vi "EdgeDetect_Camera.vi"(5 "did":string="aa5f5cb08903b53f224287e0", 7 "wid":string="e1f73355bdbd9a727fdd999e", 9 "eid":string, 11 "Scaling Factor":dbl) -> (4 "Device Out":T2, 6 "Comm":T1, 8 "image 2":picture, 15 "error out":errorcluster)   [LabVIEW 2019]
uses:
  <userlib>/Onshape/_SubVI/Cluster.ctl
  <userlib>/IoT Devices/_subVIs/HTTPComm.ctl
  <userlib>/Onshape/_SubVI/z did wid and eid.vi
  <userlib>/OnshapeFeatureFunctions/Onshape Feature Funcrions/_SubVI/FS Sketch Polyline.vi
  <userlib>/OnshapeFeatureFunctions/Onshape Feature Funcrions/_SubVI/FS Operation Extrude.vi
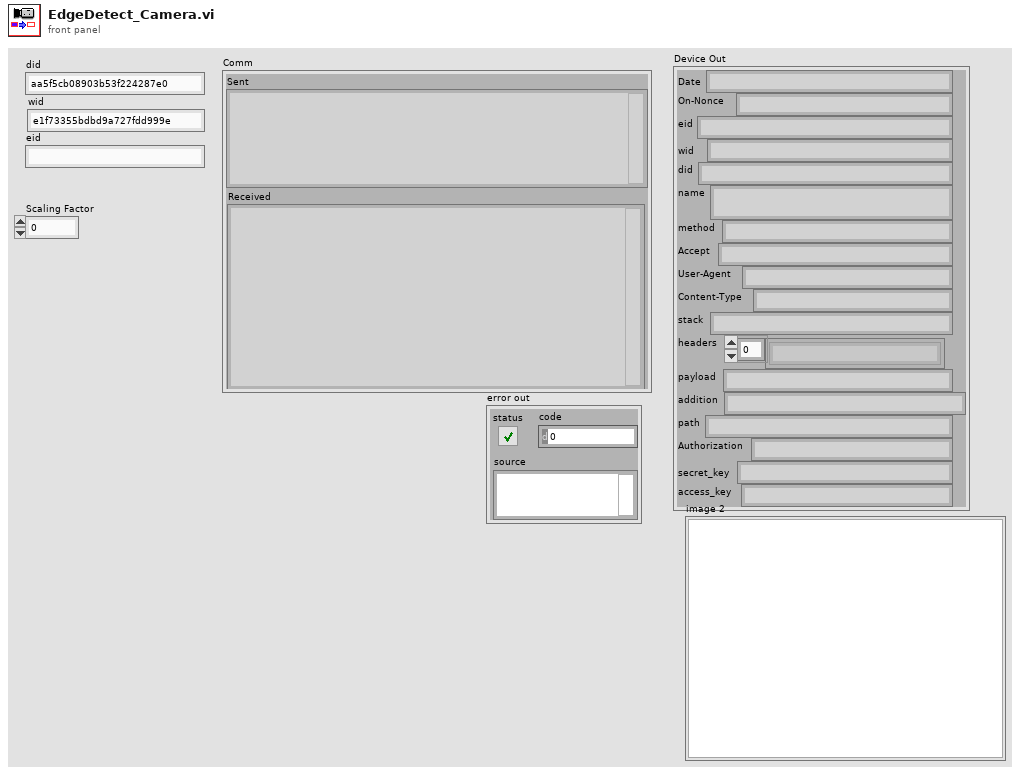
[diagram p1: front panel]
types:
  T1 = typedef "HTTPComm.ctl" = cluster{"url":string, "sent headers":string, "sent body":string, "headers":string, "body":string, "Sent":string, "Received":string}
  T2 = typedef "Cluster.ctl" = cluster{"Date":string, "On-Nonce":string, "eid":string, "wid":string, "did":string, "name":string, "method":string, "Accept":string, "User-Agent":string, "Content-Type":string, "stack":string, "headers":string[], "payload":string, "addition":string, "path":string, "Authorization":string, "secret_key":string, "access_key":string}
  T3 = typedef "QT_Image.ctl" = cluster{"Width":i32, "Height":i32, "Depth":i32, "data":u8[], "Compressed data":u8[], "Color table":u32[], "Duration":i32, "Options":i32, "Timestamp":i32, "ID":i32, "Reserved":i32, "Dialogs":u32}
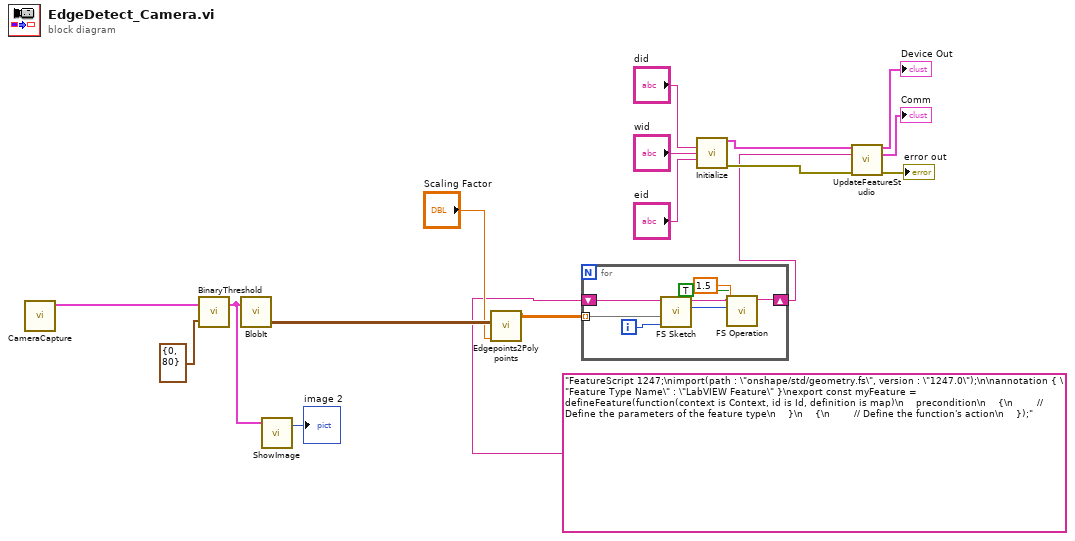
[diagram p0: block diagram]
diagram:
  n1 = call <userlib>:"CameraCapture.vi"() -> ("Image  out"=w4:T3)  [unwired: 11 in]
  n2 = call <userlib>:"BinaryThreshold.vi"("threshold"=cluster{u8, u8} {0, 80}, "Image In"=w4) -> ("Image Out"=w6:T3)  [unwired: 1 in]
  n3 = call <userlib>:"BlobIt.vi"("Image in"=w6) -> ("Array 2"=w17:cluster{"Row":i32, "Col":i32}[][])  [unwired: 1 in, 2 out]
  n4 = call <userlib>:"ShowImage.vi"("Image"=w6) -> ("image"=→"image 2":picture)  [unwired: 2 in, 1 out]
  n5 = call <userlib>:"Edgepoints2Polypoints.vi"("Scaling Factor"="Scaling Factor", "Edgepoints In"=w17) -> ("Polyline Out"=w2:dbl[][][])  [unwired: 9 in]
  n6 = for {
    tunnel: w2 -> [w24] mode=indexing
    shift-right: [w21] -> w1
    shift-left: "FeatureScript 1247;\nimport(path : \"onshape/std/geometry.fs\", version : \"1247.0\");\n\nannotation { \"Feature Type Name\" : \"LabVIEW Feature\" }\nexport const myFeature = defineFeature(function(context is Context, id is Id, definition is map)\n    precondition\n    {\n        // Define the parameters of the feature type\n    }\n    {\n        // Define the function's action\n    });" ("Feature In") -> [w23]
    i -> [w18]
    n7 = call-poly <userlib>:"FS Sketch.vi"("Sketch #"=w18, "Polyline Points"=w24, "Feature In"=w23) -> ("Feature Out"=w22:string)  [unwired: 8 in]
    n8 = call-poly <userlib>:"FS Operation.vi"("Ignore Inner Loops?"=TRUE, "Extrude Depth"=1.5, "Sketch # to Extrude"=w18, "Feature In"=w22) -> ("Feature Out"=w21:string)  [unwired: 7 in]
  }
  n9 = call-poly <userlib>:"Initialize.vi"("did"="did", "wid"="wid", "eid"="eid") -> ("Device Out"=w13:T2, "error out"=w7:errorcluster)  [unwired: 11 in]
  n10 = call <userlib>:"UpdateFeatureStudio.vi"("Device In"=w13, "FeatureScript"=w1, "error in"=w7) -> ("Device Out"=→"Device Out":T2, "Comm"=→"Comm":T1, "error out"=→"error out":errorcluster)  [unwired: 10 in]
